vi "Big Variant Cluster.vi"(1 "Cluster":T1={"Variant"=variant(u32 0), "Variant 2"=variant(u32 0), "Variant 3"=variant(u32 0), "Variant 4"=variant(u32 0), "Variant 5"=variant(u32 0), "Variant 6"=variant(u32 0), "Variant 7"=variant(u32 0), "Variant 8"=variant(u32 0), "Variant 9"=variant(u32 0), "Variant 10"=variant(u32 0), "Variant 11"=variant(u32 0), "Variant 12"=variant(u32 0), "Variant 13"=variant(u32 0), "Variant 14"=variant(u32 0), "Variant 15"=variant(u32 0), "Variant 16"=variant(u32 0), "Variant 17"=variant(u32 0), "Variant 18"=variant(u32 0), "Variant 19"=variant(u32 0), "Variant 20"=variant(u32 0), "Variant 21"=variant(u32 0), "Variant 22"=variant(u32 0), "Variant 23"=variant(u32 0), "Variant 24"=variant(u32 0), "Variant 25"=variant(u32 0), "Variant 26"=variant(u32 0), "Variant 27"=variant(u32 0), "Variant 28"=variant(u32 0), "Variant 29"=variant(u32 0), "Variant 30"=variant(u32 0), "Variant 31"=variant(u32 0), "Variant 32"=variant(u32 0), "Variant 33"=variant(u32 0), "Variant 34"=variant(u32 0), "Variant 35"=variant(u32 0), "Variant 36"=variant(u32 0), "Variant 37"=variant(u32 0), "Variant 38"=variant(u32 0), "Variant 39"=variant(u32 0), "Variant 40"=variant(u32 0), "Variant 41"=variant(u32 0), "Variant 42"=variant(u32 0), "Variant 43"=variant(u32 0), "Variant 44"=variant(u32 0), "Variant 45"=variant(u32 0), "Variant 46"=variant(u32 0), "Variant 47"=variant(u32 0), "Variant 48"=variant(u32 0), "Variant 49"=variant(u32 0), "Variant 50"=variant(u32 0), "Variant 51"=variant(u32 0), "Variant 52"=variant(u32 0), "Variant 53"=variant(u32 0), "Variant 54"=variant(u32 0), "Variant 55"=variant(u32 0), "Variant 56"=variant(u32 0), "Variant 57"=variant(u32 0), "Variant 58"=variant(u32 0), "Variant 59"=variant(u32 0), "Variant 60"=variant(u32 0), "Variant 61"=variant(u32 0), "Variant 62"=variant(u32 0), "Variant 63"=variant(u32 0), "Variant 64"=variant(u32 0), "Variant 65"=variant(u32 0), "Variant 66"=variant(u32 0), "Variant 67"=variant(u32 0), "Variant 68"=variant(u32 0), "Variant 69"=variant(u32 0), "Variant 70"=variant(u32 0), "Variant 71"=variant(u32 0), "Variant 72"=variant(u32 0), "Variant 73"=variant(u32 0), "Variant 74"=variant(u32 0), "Variant 75"=variant(u32 0), "Variant 76"=variant(u32 0), "Variant 77"=variant(u32 0), "Variant 78"=variant(u32 0), "Variant 79"=variant(u32 0), "Variant 80"=variant(u32 0), "Variant 81"=variant(u32 0), "Variant 82"=variant(u32 0), "Variant 83"=variant(u32 0), "Variant 84"=variant(u32 0), "Variant 85"=variant(u32 0), "Variant 86"=variant(u32 0), "Variant 87"=variant(u32 0), "Variant 88"=variant(u32 0), "Variant 89"=variant(u32 0), "Variant 90"=variant(u32 0), "Variant 91"=variant(u32 0), "Variant 92"=variant(u32 0), "Variant 93"=variant(u32 0), "Variant 94"=variant(u32 0), "Variant 95"=variant(u32 0), "Variant 96"=variant(u32 0), "Variant 97"=variant(u32 0), "Variant 98"=variant(u32 0), "Variant 99"=variant(u32 0), "Variant 100"=variant(u32 0), "Variant 101"=variant(u32 0), "Variant 102"=variant(u32 0), "Variant 103"=variant(u32 0), "Variant 104"=variant(u32 0), "Variant 105"=variant(u32 0), "Variant 106"=variant(u32 0), "Variant 107"=variant(u32 0), "Variant 108"=variant(u32 0), "Variant 109"=variant(u32 0), "Variant 110"=variant(u32 0), "Variant 111"=variant(u32 0), "Variant 112"=variant(u32 0), "Variant 113"=variant(u32 0), "Variant 114"=variant(u32 0), "Variant 115"=variant(u32 0), "Variant 116"=variant(u32 0), "Variant 117"=variant(u32 0), "Variant 118"=variant(u32 0), "Variant 119"=variant(u32 0), "Variant 120"=variant(u32 0), "Variant 121"=variant(u32 0), "Variant 122"=variant(u32 0), "Variant 123"=variant(u32 0), "Variant 124"=variant(u32 0), "Variant 125"=variant(u32 0), "Variant 126"=variant(u32 0), "Variant 127"=variant(u32 0), "Variant 128"=variant(u32 0), "Variant 129"=variant(u32 0), "Variant 130"=variant(u32 0), "Variant 131"=variant(u32 0), "Variant 132"=variant(u32 0), "Variant 133"=variant(u32 0), "Variant 134"=variant(u32 0), "Variant 135"=variant(u32 0), "Variant 136"=variant(u32 0), "Variant 137"=variant(u32 0), "Variant 138"=variant(u32 0), "Variant 139"=variant(u32 0), "Variant 140"=variant(u32 0), "Variant 141"=variant(u32 0), "Variant 142"=variant(u32 0), "Variant 143"=variant(u32 0), "Variant 144"=variant(u32 0), "Variant 145"=variant(u32 0), "Variant 146"=variant(u32 0), "Variant 147"=variant(u32 0), "Variant 148"=variant(u32 0), "Variant 149"=variant(u32 0), "Variant 150"=variant(u32 0), "Variant 151"=variant(u32 0), "Variant 152"=variant(u32 0), "Variant 153"=variant(u32 0), "Variant 154"=variant(u32 0), "Variant 155"=variant(u32 0), "Variant 156"=variant(u32 0), "Variant 157"=variant(u32 0), "Variant 158"=variant(u32 0), "Variant 159"=variant(u32 0), "Variant 160"=variant(u32 0), "Variant 161"=variant(u32 0), "Variant 162"=variant(u32 0), "Variant 163"=variant(u32 0), "Variant 164"=variant(u32 0), "Variant 165"=variant(u32 0), "Variant 166"=variant(u32 0), "Variant 167"=variant(u32 0), "Variant 168"=variant(u32 0), "Variant 169"=variant(u32 0), "Variant 170"=variant(u32 0), "Variant 171"=variant(u32 0), "Variant 172"=variant(u32 0), "Variant 173"=variant(u32 0), "Variant 174"=variant(u32 0), "Variant 175"=variant(u32 0), "Variant 176"=variant(u32 0), "Variant 177"=variant(u32 0), "Variant 178"=variant(u32 0), "Variant 179"=variant(u32 0), "Variant 180"=variant(u32 0), "Variant 181"=variant(u32 0), "Variant 182"=variant(u32 0), "Variant 183"=variant(u32 0), "Variant 184"=variant(u32 0), "Variant 185"=variant(u32 0), "Variant 186"=variant(u32 0), "Variant 187"=variant(u32 0), "Variant 188"=variant(u32 0), "Variant 189"=variant(u32 0), "Variant 190"=variant(u32 0), "Variant 191"=variant(u32 0), "Variant 192"=variant(u32 0), "Variant 193"=variant(u32 0), "Variant 194"=variant(u32 0), "Variant 195"=variant(u32 0), "Variant 196"=variant(u32 0), "Variant 197"=variant(u32 0), "Variant 198"=variant(u32 0), "Variant 199"=variant(u32 0), "Variant 200"=variant(u32 0), "Variant 201"=variant(u32 0), "Variant 202"=variant(u32 0), "Variant 203"=variant(u32 0), "Variant 204"=variant(u32 0), "Variant 205"=variant(u32 0), "Variant 206"=variant(u32 0), "Variant 207"=variant(u32 0), "Variant 208"=variant(u32 0), "Variant 209"=variant(u32 0), "Variant 210"=variant(u32 0), "Variant 211"=variant(u32 0), "Variant 212"=variant(u32 0), "Variant 213"=variant(u32 0), "Variant 214"=variant(u32 0), "Variant 215"=variant(u32 0), "Variant 216"=variant(u32 0), "Variant 217"=variant(u32 0), "Variant 218"=variant(u32 0), "Variant 219"=variant(u32 0), "Variant 220"=variant(u32 0), "Variant 221"=variant(u32 0), "Variant 222"=variant(u32 0), "Variant 223"=variant(u32 0), "Variant 224"=variant(u32 0), "Variant 225"=variant(u32 0), "Variant 226"=variant(u32 0), "Variant 227"=variant(u32 0), "Variant 228"=variant(u32 0), "Variant 229"=variant(u32 0), "Variant 230"=variant(u32 0), "Variant 231"=variant(u32 0), "Variant 232"=variant(u32 0), "Variant 233"=variant(u32 0), "Variant 234"=variant(u32 0), "Variant 235"=variant(u32 0), "Variant 236"=variant(u32 0), "Variant 237"=variant(u32 0), "Variant 238"=variant(u32 0), "Variant 239"=variant(u32 0), "Variant 240"=variant(u32 0), "Variant 241"=variant(u32 0), "Variant 242"=variant(u32 0), "Variant 243"=variant(u32 0), "Variant 244"=variant(u32 0), "Variant 245"=variant(u32 0), "Variant 246"=variant(u32 0), "Variant 247"=variant(u32 0), "Variant 248"=variant(u32 0), "Variant 249"=variant(u32 0), "Variant 250"=variant(u32 0), "Variant 251"=variant(u32 0), "Variant 252"=variant(u32 0), "Variant 253"=variant(u32 0), "Variant 254"=variant(u32 0), "Variant 255"=variant(u32 0), "Variant 256"=variant(u32 0), "Variant 257"=variant(u32 0), "Variant 258"=variant(u32 0), "Variant 259"=variant(u32 0), "Variant 260"=variant(u32 0), "Variant 261"=variant(u32 0), "Variant 262"=variant(u32 0), "Variant 263"=variant(u32 0), "Variant 264"=variant(u32 0), "Variant 265"=variant(u32 0), "Variant 266"=variant(u32 0), "Variant 267"=variant(u32 0), "Variant 268"=variant(u32 0), "Variant 269"=variant(u32 0), "Variant 270"=variant(u32 0), "Variant 271"=variant(u32 0), "Variant 272"=variant(u32 0), "Variant 273"=variant(u32 0), "Variant 274"=variant(u32 0), "Variant 275"=variant(u32 0), "Variant 276"=variant(u32 0), "Variant 277"=variant(u32 0), "Variant 278"=variant(u32 0), "Variant 279"=variant(u32 0), "Variant 280"=variant(u32 0), "Variant 281"=variant(u32 0), "Variant 282"=variant(u32 0), "Variant 283"=variant(u32 0), "Variant 284"=variant(u32 0), "Variant 285"=variant(u32 0), "Variant 286"=variant(u32 0), "Variant 287"=variant(u32 0), "Variant 288"=variant(u32 0), "Variant 289"=variant(u32 0), "Variant 290"=variant(u32 0), "Variant 291"=variant(u32 0), "Variant 292"=variant(u32 0), "Variant 293"=variant(u32 0), "Variant 294"=variant(u32 0), "Variant 295"=variant(u32 0), "Variant 296"=variant(u32 0), "Variant 297"=variant(u32 0), "Variant 298"=variant(u32 0), "Variant 299"=variant(u32 0), "Variant 300"=variant(u32 0), "Variant 301"=variant(u32 0), "Variant 302"=variant(u32 0), "Variant 303"=variant(u32 0), "Variant 304"=variant(u32 0), "Variant 305"=variant(u32 0), "Variant 306"=variant(u32 0), "Variant 307"=variant(u32 0), "Variant 308"=variant(u32 0), "Variant 309"=variant(u32 0), "Variant 310"=variant(u32 0), "Variant 311"=variant(u32 0), "Variant 312"=variant(u32 0), "Variant 313"=variant(u32 0), "Variant 314"=variant(u32 0), "Variant 315"=variant(u32 0), "Variant 316"=variant(u32 0), "Variant 317"=variant(u32 0), "Variant 318"=variant(u32 0), "Variant 319"=variant(u32 0), "Variant 320"=variant(u32 0), "Variant 321"=variant(u32 0), "Variant 322"=variant(u32 0), "Variant 323"=variant(u32 0), "Variant 324"=variant(u32 0), "Variant 325"=variant(u32 0), "Variant 326"=variant(u32 0), "Variant 327"=variant(u32 0), "Variant 328"=variant(u32 0), "Variant 329"=variant(u32 0), "Variant 330"=variant(u32 0), "Variant 331"=variant(u32 0), "Variant 332"=variant(u32 0), "Variant 333"=variant(u32 0), "Variant 334"=variant(u32 0), "Variant 335"=variant(u32 0), "Variant 336"=variant(u32 0), "Variant 337"=variant(u32 0), "Variant 338"=variant(u32 0), "Variant 339"=variant(u32 0), "Variant 340"=variant(u32 0), "Variant 341"=variant(u32 0), "Variant 342"=variant(u32 0), "Variant 343"=variant(u32 0), "Variant 344"=variant(u32 0), "Variant 345"=variant(u32 0), "Variant 346"=variant(u32 0), "Variant 347"=variant(u32 0), "Variant 348"=variant(u32 0), "Variant 349"=variant(u32 0), "Variant 350"=variant(u32 0), "Variant 351"=variant(u32 0), "Variant 352"=variant(u32 0), "Variant 353"=variant(u32 0), "Variant 354"=variant(u32 0), "Variant 355"=variant(u32 0), "Variant 356"=variant(u32 0), "Variant 357"=variant(u32 0), "Variant 358"=variant(u32 0), "Variant 359"=variant(u32 0), "Variant 360"=variant(u32 0), "Variant 361"=variant(u32 0), "Variant 362"=variant(u32 0), "Variant 363"=variant(u32 0), "Variant 364"=variant(u32 0), "Variant 365"=variant(u32 0), "Variant 366"=variant(u32 0), "Variant 367"=variant(u32 0), "Variant 368"=variant(u32 0), "Variant 369"=variant(u32 0), "Variant 370"=variant(u32 0), "Variant 371"=variant(u32 0), "Variant 372"=variant(u32 0), "Variant 373"=variant(u32 0), "Variant 374"=variant(u32 0), "Variant 375"=variant(u32 0), "Variant 376"=variant(u32 0), "Variant 377"=variant(u32 0), "Variant 378"=variant(u32 0), "Variant 379"=variant(u32 0), "Variant 380"=variant(u32 0), "Variant 381"=variant(u32 0), "Variant 382"=variant(u32 0), "Variant 383"=variant(u32 0), "Variant 384"=variant(u32 0), "Variant 385"=variant(u32 0), "Variant 386"=variant(u32 0), "Variant 387"=variant(u32 0), "Variant 388"=variant(u32 0), "Variant 389"=variant(u32 0), "Variant 390"=variant(u32 0), "Variant 391"=variant(u32 0), "Variant 392"=variant(u32 0), "Variant 393"=variant(u32 0), "Variant 394"=variant(u32 0), "Variant 395"=variant(u32 0), "Variant 396"=variant(u32 0), "Variant 397"=variant(u32 0), "Variant 398"=variant(u32 0), "Variant 399"=variant(u32 0), "Variant 400"=variant(u32 0), "Variant 401"=variant(u32 0), "Variant 402"=variant(u32 0), "Variant 403"=variant(u32 0), "Variant 404"=variant(u32 0), "Variant 405"=variant(u32 0), "Variant 406"=variant(u32 0), "Variant 407"=variant(u32 0), "Variant 408"=variant(u32 0), "Variant 409"=variant(u32 0), "Variant 410"=variant(u32 0), "Variant 411"=variant(u32 0), "Variant 412"=variant(u32 0), "Variant 413"=variant(u32 0), "Variant 414"=variant(u32 0), "Variant 415"=variant(u32 0), "Variant 416"=variant(u32 0), "Variant 417"=variant(u32 0), "Variant 418"=variant(u32 0), "Variant 419"=variant(u32 0), "Variant 420"=variant(u32 0), "Variant 421"=variant(u32 0), "Variant 422"=variant(u32 0), "Variant 423"=variant(u32 0), "Variant 424"=variant(u32 0), "Variant 425"=variant(u32 0), "Variant 426"=variant(u32 0), "Variant 427"=variant(u32 0), "Variant 428"=variant(u32 0), "Variant 429"=variant(u32 0), "Variant 430"=variant(u32 0), "Variant 431"=variant(u32 0), "Variant 432"=variant(u32 0), "Variant 433"=variant(u32 0), "Variant 434"=variant(u32 0), "Variant 435"=variant(u32 0), "Variant 436"=variant(u32 0), "Variant 437"=variant(u32 0), "Variant 438"=variant(u32 0), "Variant 439"=variant(u32 0), "Variant 440"=variant(u32 0), "Variant 441"=variant(u32 0), "Variant 442"=variant(u32 0), "Variant 443"=variant(u32 0), "Variant 444"=variant(u32 0), "Variant 445"=variant(u32 0), "Variant 446"=variant(u32 0), "Variant 447"=variant(u32 0), "Variant 448"=variant(u32 0), "Variant 449"=variant(u32 0), "Variant 450"=variant(u32 0), "Variant 451"=variant(u32 0), "Variant 452"=variant(u32 0), "Variant 453"=variant(u32 0), "Variant 454"=variant(u32 0), "Variant 455"=variant(u32 0), "Variant 456"=variant(u32 0), "Variant 457"=variant(u32 0), "Variant 458"=variant(u32 0), "Variant 459"=variant(u32 0), "Variant 460"=variant(u32 0), "Variant 461"=variant(u32 0), "Variant 462"=variant(u32 0), "Variant 463"=variant(u32 0), "Variant 464"=variant(u32 0), "Variant 465"=variant(u32 0), "Variant 466"=variant(u32 0), "Variant 467"=variant(u32 0), "Variant 468"=variant(u32 0), "Variant 469"=variant(u32 0), "Variant 470"=variant(u32 0), "Variant 471"=variant(u32 0), "Variant 472"=variant(u32 0), "Variant 473"=variant(u32 0), "Variant 474"=variant(u32 0), "Variant 475"=variant(u32 0), "Variant 476"=variant(u32 0), "Variant 477"=variant(u32 0), "Variant 478"=variant(u32 0), "Variant 479"=variant(u32 0), "Variant 480"=variant(u32 0), "Variant 481"=variant(u32 0), "Variant 482"=variant(u32 0), "Variant 483"=variant(u32 0), "Variant 484"=variant(u32 0), "Variant 485"=variant(u32 0), "Variant 486"=variant(u32 0), "Variant 487"=variant(u32 0), "Variant 488"=variant(u32 0), "Variant 489"=variant(u32 0), "Variant 490"=variant(u32 0), "Variant 491"=variant(u32 0), "Variant 492"=variant(u32 0), "Variant 493"=variant(u32 0), "Variant 494"=variant(u32 0), "Variant 495"=variant(u32 0), "Variant 496"=variant(u32 0), "Variant 497"=variant(u32 0), "Variant 498"=variant(u32 0), "Variant 499"=variant(u32 0), "Variant 500"=variant(u32 0), "Variant 501"=variant(u32 0), "Variant 502"=variant(u32 0), "Variant 503"=variant(u32 0), "Variant 504"=variant(u32 0), "Variant 505"=variant(u32 0), "Variant 506"=variant(u32 0), "Variant 507"=variant(u32 0), "Variant 508"=variant(u32 0), "Variant 509"=variant(u32 0), "Variant 510"=variant(u32 0), "Variant 511"=variant(u32 0), "Variant 512"=variant(u32 0), "Variant 513"=variant(u32 0), "Variant 514"=variant(u32 0), "Variant 515"=variant(u32 0), "Variant 516"=variant(u32 0), "Variant 517"=variant(u32 0), "Variant 518"=variant(u32 0), "Variant 519"=variant(u32 0), "Variant 520"=variant(u32 0), "Variant 521"=variant(u32 0), "Variant 522"=variant(u32 0), "Variant 523"=variant(u32 0), "Variant 524"=variant(u32 0), "Variant 525"=variant(u32 0), "Variant 526"=variant(u32 0), "Variant 527"=variant(u32 0), "Variant 528"=variant(u32 0), "Variant 529"=variant(u32 0), "Variant 530"=variant(u32 0), "Variant 531"=variant(u32 0), "Variant 532"=variant(u32 0), "Variant 533"=variant(u32 0), "Variant 534"=variant(u32 0), "Variant 535"=variant(u32 0), "Variant 536"=variant(u32 0), "Variant 537"=variant(u32 0), "Variant 538"=variant(u32 0), "Variant 539"=variant(u32 0), "Variant 540"=variant(u32 0), "Variant 541"=variant(u32 0), "Variant 542"=variant(u32 0), "Variant 543"=variant(u32 0), "Variant 544"=variant(u32 0), "Variant 545"=variant(u32 0), "Variant 546"=variant(u32 0), "Variant 547"=variant(u32 0), "Variant 548"=variant(u32 0), "Variant 549"=variant(u32 0), "Variant 550"=variant(u32 0), "Variant 551"=variant(u32 0), "Variant 552"=variant(u32 0), "Variant 553"=variant(u32 0), "Variant 554"=variant(u32 0), "Variant 555"=variant(u32 0), "Variant 556"=variant(u32 0), "Variant 557"=variant(u32 0), "Variant 558"=variant(u32 0), "Variant 559"=variant(u32 0), "Variant 560"=variant(u32 0), "Variant 561"=variant(u32 0), "Variant 562"=variant(u32 0), "Variant 563"=variant(u32 0), "Variant 564"=variant(u32 0), "Variant 565"=variant(u32 0), "Variant 566"=variant(u32 0), "Variant 567"=variant(u32 0), "Variant 568"=variant(u32 0), "Variant 569"=variant(u32 0), "Variant 570"=variant(u32 0), "Variant 571"=variant(u32 0), "Variant 572"=variant(u32 0), "Variant 573"=variant(u32 0), "Variant 574"=variant(u32 0), "Variant 575"=variant(u32 0), "Variant 576"=variant(u32 0), "Variant 577"=variant(u32 0), "Variant 578"=variant(u32 0), "Variant 579"=variant(u32 0), "Variant 580"=variant(u32 0), "Variant 581"=variant(u32 0), "Variant 582"=variant(u32 0), "Variant 583"=variant(u32 0), "Variant 584"=variant(u32 0), "Variant 585"=variant(u32 0), "Variant 586"=variant(u32 0), "Variant 587"=variant(u32 0), "Variant 588"=variant(u32 0), "Variant 589"=variant(u32 0), "Variant 590"=variant(u32 0), "Variant 591"=variant(u32 0), "Variant 592"=variant(u32 0), "Variant 593"=variant(u32 0), "Variant 594"=variant(u32 0), "Variant 595"=variant(u32 0), "Variant 596"=variant(u32 0), "Variant 597"=variant(u32 0), "Variant 598"=variant(u32 0), "Variant 599"=variant(u32 0), "Variant 600"=variant(u32 0), "Variant 601"=variant(u32 0), "Variant 602"=variant(u32 0), "Variant 603"=variant(u32 0), "Variant 604"=variant(u32 0), "Variant 605"=variant(u32 0), "Variant 606"=variant(u32 0), "Variant 607"=variant(u32 0), "Variant 608"=variant(u32 0), "Variant 609"=variant(u32 0), "Variant 610"=variant(u32 0), "Variant 611"=variant(u32 0), "Variant 612"=variant(u32 0), "Variant 613"=variant(u32 0), "Variant 614"=variant(u32 0), "Variant 615"=variant(u32 0), "Variant 616"=variant(u32 0), "Variant 617"=variant(u32 0), "Variant 618"=variant(u32 0), "Variant 619"=variant(u32 0), "Variant 620"=variant(u32 0), "Variant 621"=variant(u32 0), "Variant 622"=variant(u32 0), "Variant 623"=variant(u32 0), "Variant 624"=variant(u32 0), "Variant 625"=variant(u32 0), "Variant 626"=variant(u32 0), "Variant 627"=variant(u32 0), "Variant 628"=variant(u32 0), "Variant 629"=variant(u32 0), "Variant 630"=variant(u32 0), "Variant 631"=variant(u32 0), "Variant 632"=variant(u32 0), "Variant 633"=variant(u32 0), "Variant 634"=variant(u32 0), "Variant 635"=variant(u32 0), "Variant 636"=variant(u32 0), "Variant 637"=variant(u32 0), "Variant 638"=variant(u32 0), "Variant 639"=variant(u32 0), "Variant 640"=variant(u32 0), "Variant 641"=variant(u32 0), "Variant 642"=variant(u32 0), "Variant 643"=variant(u32 0), "Variant 644"=variant(u32 0), "Variant 645"=variant(u32 0), "Variant 646"=variant(u32 0), "Variant 647"=variant(u32 0), "Variant 648"=variant(u32 0), "Variant 649"=variant(u32 0), "Variant 650"=variant(u32 0), "Variant 651"=variant(u32 0), "Variant 652"=variant(u32 0), "Variant 653"=variant(u32 0), "Variant 654"=variant(u32 0), "Variant 655"=variant(u32 0), "Variant 656"=variant(u32 0), "Variant 657"=variant(u32 0), "Variant 658"=variant(u32 0), "Variant 659"=variant(u32 0), "Variant 660"=variant(u32 0), "Variant 661"=variant(u32 0), "Variant 662"=variant(u32 0), "Variant 663"=variant(u32 0), "Variant 664"=variant(u32 0), "Variant 665"=variant(u32 0), "Variant 666"=variant(u32 0), "Variant 667"=variant(u32 0), "Variant 668"=variant(u32 0), "Variant 669"=variant(u32 0), "Variant 670"=variant(u32 0), "Variant 671"=variant(u32 0), "Variant 672"=variant(u32 0), "Variant 673"=variant(u32 0), "Variant 674"=variant(u32 0), "Variant 675"=variant(u32 0), "Variant 676"=variant(u32 0), "Variant 677"=variant(u32 0), "Variant 678"=variant(u32 0), "Variant 679"=variant(u32 0), "Variant 680"=variant(u32 0), "Variant 681"=variant(u32 0), "Variant 682"=variant(u32 0), "Variant 683"=variant(u32 0), "Variant 684"=variant(u32 0), "Variant 685"=variant(u32 0), "Variant 686"=variant(u32 0), "Variant 687"=variant(u32 0), "Variant 688"=variant(u32 0), "Variant 689"=variant(u32 0), "Variant 690"=variant(u32 0), "Variant 691"=variant(u32 0), "Variant 692"=variant(u32 0), "Variant 693"=variant(u32 0), "Variant 694"=variant(u32 0), "Variant 695"=variant(u32 0), "Variant 696"=variant(u32 0), "Variant 697"=variant(u32 0), "Variant 698"=variant(u32 0), "Variant 699"=variant(u32 0), "Variant 700"=variant(u32 0), "Variant 701"=variant(u32 0), "Variant 702"=variant(u32 0), "Variant 703"=variant(u32 0), "Variant 704"=variant(u32 0), "Variant 705"=variant(u32 0), "Variant 706"=variant(u32 0), "Variant 707"=variant(u32 0), "Variant 708"=variant(u32 0), "Variant 709"=variant(u32 0), "Variant 710"=variant(u32 0), "Variant 711"=variant(u32 0), "Variant 712"=variant(u32 0), "Variant 713"=variant(u32 0), "Variant 714"=variant(u32 0), "Variant 715"=variant(u32 0), "Variant 716"=variant(u32 0), "Variant 717"=variant(u32 0), "Variant 718"=variant(u32 0), "Variant 719"=variant(u32 0), "Variant 720"=variant(u32 0), "Variant 721"=variant(u32 0), "Variant 722"=variant(u32 0), "Variant 723"=variant(u32 0), "Variant 724"=variant(u32 0), "Variant 725"=variant(u32 0), "Variant 726"=variant(u32 0), "Variant 727"=variant(u32 0), "Variant 728"=variant(u32 0), "Variant 729"=variant(u32 0), "Variant 730"=variant(u32 0), "Variant 731"=variant(u32 0), "Variant 732"=variant(u32 0), "Variant 733"=variant(u32 0), "Variant 734"=variant(u32 0), "Variant 735"=variant(u32 0), "Variant 736"=variant(u32 0), "Variant 737"=variant(u32 0), "Variant 738"=variant(u32 0), "Variant 739"=variant(u32 0), "Variant 740"=variant(u32 0), "Variant 741"=variant(u32 0), "Variant 742"=variant(u32 0), "Variant 743"=variant(u32 0), "Variant 744"=variant(u32 0), "Variant 745"=variant(u32 0), "Variant 746"=variant(u32 0), "Variant 747"=variant(u32 0), "Variant 748"=variant(u32 0), "Variant 749"=variant(u32 0), "Variant 750"=variant(u32 0), "Variant 751"=variant(u32 0), "Variant 752"=variant(u32 0), "Variant 753"=variant(u32 0), "Variant 754"=variant(u32 0), "Variant 755"=variant(u32 0), "Variant 756"=variant(u32 0), "Variant 757"=variant(u32 0), "Variant 758"=variant(u32 0), "Variant 759"=variant(u32 0), "Variant 760"=variant(u32 0), "Variant 761"=variant(u32 0), "Variant 762"=variant(u32 0), "Variant 763"=variant(u32 0), "Variant 764"=variant(u32 0), "Variant 765"=variant(u32 0), "Variant 766"=variant(u32 0), "Variant 767"=variant(u32 0), "Variant 768"=variant(u32 0), "Variant 769"=variant(u32 0), "Variant 770"=variant(u32 0), "Variant 771"=variant(u32 0), "Variant 772"=variant(u32 0), "Variant 773"=variant(u32 0), "Variant 774"=variant(u32 0), "Variant 775"=variant(u32 0), "Variant 776"=variant(u32 0), "Variant 777"=variant(u32 0), "Variant 778"=variant(u32 0), "Variant 779"=variant(u32 0), "Variant 780"=variant(u32 0), "Variant 781"=variant(u32 0), "Variant 782"=variant(u32 0), "Variant 783"=variant(u32 0), "Variant 784"=variant(u32 0), "Variant 785"=variant(u32 0), "Variant 786"=variant(u32 0), "Variant 787"=variant(u32 0), "Variant 788"=variant(u32 0), "Variant 789"=variant(u32 0), "Variant 790"=variant(u32 0), "Variant 791"=variant(u32 0), "Variant 792"=variant(u32 0), "Variant 793"=variant(u32 0), "Variant 794"=variant(u32 0), "Variant 795"=variant(u32 0), "Variant 796"=variant(u32 0), "Variant 797"=variant(u32 0), "Variant 798"=variant(u32 0), "Variant 799"=variant(u32 0), "Variant 800"=variant(u32 0), "Variant 801"=variant(u32 0), "Variant 802"=variant(u32 0), "Variant 803"=variant(u32 0), "Variant 804"=variant(u32 0), "Variant 805"=variant(u32 0), "Variant 806"=variant(u32 0), "Variant 807"=variant(u32 0), "Variant 808"=variant(u32 0), "Variant 809"=variant(u32 0), "Variant 810"=variant(u32 0), "Variant 811"=variant(u32 0), "Variant 812"=variant(u32 0), "Variant 813"=variant(u32 0), "Variant 814"=variant(u32 0), "Variant 815"=variant(u32 0), "Variant 816"=variant(u32 0), "Variant 817"=variant(u32 0), "Variant 818"=variant(u32 0), "Variant 819"=variant(u32 0), "Variant 820"=variant(u32 0), "Variant 821"=variant(u32 0), "Variant 822"=variant(u32 0), "Variant 823"=variant(u32 0), "Variant 824"=variant(u32 0), "Variant 825"=variant(u32 0), "Variant 826"=variant(u32 0), "Variant 827"=variant(u32 0), "Variant 828"=variant(u32 0), "Variant 829"=variant(u32 0), "Variant 830"=variant(u32 0), "Variant 831"=variant(u32 0), "Variant 832"=variant(u32 0), "Variant 833"=variant(u32 0), "Variant 834"=variant(u32 0), "Variant 835"=variant(u32 0), "Variant 836"=variant(u32 0), "Variant 837"=variant(u32 0), "Variant 838"=variant(u32 0), "Variant 839"=variant(u32 0), "Variant 840"=variant(u32 0), "Variant 841"=variant(u32 0), "Variant 842"=variant(u32 0), "Variant 843"=variant(u32 0), "Variant 844"=variant(u32 0), "Variant 845"=variant(u32 0), "Variant 846"=variant(u32 0), "Variant 847"=variant(u32 0), "Variant 848"=variant(u32 0), "Variant 849"=variant(u32 0), "Variant 850"=variant(u32 0), "Variant 851"=variant(u32 0), "Variant 852"=variant(u32 0), "Variant 853"=variant(u32 0), "Variant 854"=variant(u32 0), "Variant 855"=variant(u32 0), "Variant 856"=variant(u32 0), "Variant 857"=variant(u32 0), "Variant 858"=variant(u32 0), "Variant 859"=variant(u32 0), "Variant 860"=variant(u32 0), "Variant 861"=variant(u32 0), "Variant 862"=variant(u32 0), "Variant 863"=variant(u32 0), "Variant 864"=variant(u32 0), "Variant 865"=variant(u32 0), "Variant 866"=variant(u32 0), "Variant 867"=variant(u32 0), "Variant 868"=variant(u32 0), "Variant 869"=variant(u32 0), "Variant 870"=variant(u32 0), "Variant 871"=variant(u32 0), "Variant 872"=variant(u32 0), "Variant 873"=variant(u32 0), "Variant 874"=variant(u32 0), "Variant 875"=variant(u32 0), "Variant 876"=variant(u32 0), "Variant 877"=variant(u32 0), "Variant 878"=variant(u32 0), "Variant 879"=variant(u32 0), "Variant 880"=variant(u32 0), "Variant 881"=variant(u32 0), "Variant 882"=variant(u32 0), "Variant 883"=variant(u32 0), "Variant 884"=variant(u32 0), "Variant 885"=variant(u32 0), "Variant 886"=variant(u32 0), "Variant 887"=variant(u32 0), "Variant 888"=variant(u32 0), "Variant 889"=variant(u32 0), "Variant 890"=variant(u32 0), "Variant 891"=variant(u32 0), "Variant 892"=variant(u32 0), "Variant 893"=variant(u32 0), "Variant 894"=variant(u32 0), "Variant 895"=variant(u32 0), "Variant 896"=variant(u32 0), "Variant 897"=variant(u32 0), "Variant 898"=variant(u32 0), "Variant 899"=variant(u32 0), "Variant 900"=variant(u32 0), "Variant 901"=variant(u32 0), "Variant 902"=variant(u32 0), "Variant 903"=variant(u32 0), "Variant 904"=variant(u32 0), "Variant 905"=variant(u32 0), "Variant 906"=variant(u32 0), "Variant 907"=variant(u32 0), "Variant 908"=variant(u32 0), "Variant 909"=variant(u32 0), "Variant 910"=variant(u32 0), "Variant 911"=variant(u32 0), "Variant 912"=variant(u32 0), "Variant 913"=variant(u32 0), "Variant 914"=variant(u32 0), "Variant 915"=variant(u32 0), "Variant 916"=variant(u32 0), "Variant 917"=variant(u32 0), "Variant 918"=variant(u32 0), "Variant 919"=variant(u32 0), "Variant 920"=variant(u32 0), "Variant 921"=variant(u32 0), "Variant 922"=variant(u32 0), "Variant 923"=variant(u32 0), "Variant 924"=variant(u32 0), "Variant 925"=variant(u32 0), "Variant 926"=variant(u32 0), "Variant 927"=variant(u32 0), "Variant 928"=variant(u32 0), "Variant 929"=variant(u32 0), "Variant 930"=variant(u32 0), "Variant 931"=variant(u32 0), "Variant 932"=variant(u32 0), "Variant 933"=variant(u32 0), "Variant 934"=variant(u32 0), "Variant 935"=variant(u32 0), "Variant 936"=variant(u32 0), "Variant 937"=variant(u32 0), "Variant 938"=variant(u32 0), "Variant 939"=variant(u32 0), "Variant 940"=variant(u32 0), "Variant 941"=variant(u32 0), "Variant 942"=variant(u32 0), "Variant 943"=variant(u32 0), "Variant 944"=variant(u32 0), "Variant 945"=variant(u32 0), "Variant 946"=variant(u32 0), "Variant 947"=variant(u32 0), "Variant 948"=variant(u32 0), "Variant 949"=variant(u32 0), "Variant 950"=variant(u32 0), "Variant 951"=variant(u32 0), "Variant 952"=variant(u32 0), "Variant 953"=variant(u32 0), "Variant 954"=variant(u32 0), "Variant 955"=variant(u32 0), "Variant 956"=variant(u32 0), "Variant 957"=variant(u32 0), "Variant 958"=variant(u32 0), "Variant 959"=variant(u32 0), "Variant 960"=variant(u32 0), "Variant 961"=variant(u32 0), "Variant 962"=variant(u32 0), "Variant 963"=variant(u32 0), "Variant 964"=variant(u32 0), "Variant 965"=variant(u32 0), "Variant 966"=variant(u32 0), "Variant 967"=variant(u32 0), "Variant 968"=variant(u32 0), "Variant 969"=variant(u32 0), "Variant 970"=variant(u32 0), "Variant 971"=variant(u32 0), "Variant 972"=variant(u32 0), "Variant 973"=variant(u32 0), "Variant 974"=variant(u32 0), "Variant 975"=variant(u32 0), "Variant 976"=variant(u32 0), "Variant 977"=variant(u32 0), "Variant 978"=variant(u32 0), "Variant 979"=variant(u32 0), "Variant 980"=variant(u32 0), "Variant 981"=variant(u32 0), "Variant 982"=variant(u32 0), "Variant 983"=variant(u32 0), "Variant 984"=variant(u32 0), "Variant 985"=variant(u32 0), "Variant 986"=variant(u32 0), "Variant 987"=variant(u32 0), "Variant 988"=variant(u32 0), "Variant 989"=variant(u32 0), "Variant 990"=variant(u32 0), "Variant 991"=variant(u32 0), "Variant 992"=variant(u32 0), "Variant 993"=variant(u32 0), "Variant 994"=variant(u32 0), "Variant 995"=variant(u32 0), "Variant 996"=variant(u32 0), "Variant 997"=variant(u32 0), "Variant 998"=variant(u32 0), "Variant 999"=variant(u32 0), "Variant 1000"=variant(u32 123)}) -> (0 "Cluster 2":T1)   [LabVIEW 2012]
types:
  T1 = cluster{"Variant":variant, "Variant 2":variant, "Variant 3":variant, "Variant 4":variant, "Variant 5":variant, "Variant 6":variant, "Variant 7":variant, "Variant 8":variant, "Variant 9":variant, "Variant 10":variant, "Variant 11":variant, "Variant 12":variant, "Variant 13":variant, "Variant 14":variant, "Variant 15":variant, "Variant 16":variant, "Variant 17":variant, "Variant 18":variant, "Variant 19":variant, "Variant 20":variant, "Variant 21":variant, "Variant 22":variant, "Variant 23":variant, "Variant 24":variant, "Variant 25":variant, "Variant 26":variant, "Variant 27":variant, "Variant 28":variant, "Variant 29":variant, "Variant 30":variant, "Variant 31":variant, "Variant 32":variant, "Variant 33":variant, "Variant 34":variant, "Variant 35":variant, "Variant 36":variant, "Variant 37":variant, "Variant 38":variant, "Variant 39":variant, "Variant 40":variant, "Variant 41":variant, "Variant 42":variant, "Variant 43":variant, "Variant 44":variant, "Variant 45":variant, "Variant 46":variant, "Variant 47":variant, "Variant 48":variant, "Variant 49":variant, "Variant 50":variant, "Variant 51":variant, "Variant 52":variant, "Variant 53":variant, "Variant 54":variant, "Variant 55":variant, "Variant 56":variant, "Variant 57":variant, "Variant 58":variant, "Variant 59":variant, "Variant 60":variant, "Variant 61":variant, "Variant 62":variant, "Variant 63":variant, "Variant 64":variant, "Variant 65":variant, "Variant 66":variant, "Variant 67":variant, "Variant 68":variant, "Variant 69":variant, "Variant 70":variant, "Variant 71":variant, "Variant 72":variant, "Variant 73":variant, "Variant 74":variant, "Variant 75":variant, "Variant 76":variant, "Variant 77":variant, "Variant 78":variant, "Variant 79":variant, "Variant 80":variant, "Variant 81":variant, "Variant 82":variant, "Variant 83":variant, "Variant 84":variant, "Variant 85":variant, "Variant 86":variant, "Variant 87":variant, "Variant 88":variant, "Variant 89":variant, "Variant 90":variant, "Variant 91":variant, "Variant 92":variant, "Variant 93":variant, "Variant 94":variant, "Variant 95":variant, "Variant 96":variant, "Variant 97":variant, "Variant 98":variant, "Variant 99":variant, "Variant 100":variant, "Variant 101":variant, "Variant 102":variant, "Variant 103":variant, "Variant 104":variant, "Variant 105":variant, "Variant 106":variant, "Variant 107":variant, "Variant 108":variant, "Variant 109":variant, "Variant 110":variant, "Variant 111":variant, "Variant 112":variant, "Variant 113":variant, "Variant 114":variant, "Variant 115":variant, "Variant 116":variant, "Variant 117":variant, "Variant 118":variant, "Variant 119":variant, "Variant 120":variant, "Variant 121":variant, "Variant 122":variant, "Variant 123":variant, "Variant 124":variant, "Variant 125":variant, "Variant 126":variant, "Variant 127":variant, "Variant 128":variant, "Variant 129":variant, "Variant 130":variant, "Variant 131":variant, "Variant 132":variant, "Variant 133":variant, "Variant 134":variant, "Variant 135":variant, "Variant 136":variant, "Variant 137":variant, "Variant 138":variant, "Variant 139":variant, "Variant 140":variant, "Variant 141":variant, "Variant 142":variant, "Variant 143":variant, "Variant 144":variant, "Variant 145":variant, "Variant 146":variant, "Variant 147":variant, "Variant 148":variant, "Variant 149":variant, "Variant 150":variant, "Variant 151":variant, "Variant 152":variant, "Variant 153":variant, "Variant 154":variant, "Variant 155":variant, "Variant 156":variant, "Variant 157":variant, "Variant 158":variant, "Variant 159":variant, "Variant 160":variant, "Variant 161":variant, "Variant 162":variant, "Variant 163":variant, "Variant 164":variant, "Variant 165":variant, "Variant 166":variant, "Variant 167":variant, "Variant 168":variant, "Variant 169":variant, "Variant 170":variant, "Variant 171":variant, "Variant 172":variant, "Variant 173":variant, "Variant 174":variant, "Variant 175":variant, "Variant 176":variant, "Variant 177":variant, "Variant 178":variant, "Variant 179":variant, "Variant 180":variant, "Variant 181":variant, "Variant 182":variant, "Variant 183":variant, "Variant 184":variant, "Variant 185":variant, "Variant 186":variant, "Variant 187":variant, "Variant 188":variant, "Variant 189":variant, "Variant 190":variant, "Variant 191":variant, "Variant 192":variant, "Variant 193":variant, "Variant 194":variant, "Variant 195":variant, "Variant 196":variant, "Variant 197":variant, "Variant 198":variant, "Variant 199":variant, "Variant 200":variant, "Variant 201":variant, "Variant 202":variant, "Variant 203":variant, "Variant 204":variant, "Variant 205":variant, "Variant 206":variant, "Variant 207":variant, "Variant 208":variant, "Variant 209":variant, "Variant 210":variant, "Variant 211":variant, "Variant 212":variant, "Variant 213":variant, "Variant 214":variant, "Variant 215":variant, "Variant 216":variant, "Variant 217":variant, "Variant 218":variant, "Variant 219":variant, "Variant 220":variant, "Variant 221":variant, "Variant 222":variant, "Variant 223":variant, "Variant 224":variant, "Variant 225":variant, "Variant 226":variant, "Variant 227":variant, "Variant 228":variant, "Variant 229":variant, "Variant 230":variant, "Variant 231":variant, "Variant 232":variant, "Variant 233":variant, "Variant 234":variant, "Variant 235":variant, "Variant 236":variant, "Variant 237":variant, "Variant 238":variant, "Variant 239":variant, "Variant 240":variant, "Variant 241":variant, "Variant 242":variant, "Variant 243":variant, "Variant 244":variant, "Variant 245":variant, "Variant 246":variant, "Variant 247":variant, "Variant 248":variant, "Variant 249":variant, "Variant 250":variant, "Variant 251":variant, "Variant 252":variant, "Variant 253":variant, "Variant 254":variant, "Variant 255":variant, "Variant 256":variant, "Variant 257":variant, "Variant 258":variant, "Variant 259":variant, "Variant 260":variant, "Variant 261":variant, "Variant 262":variant, "Variant 263":variant, "Variant 264":variant, "Variant 265":variant, "Variant 266":variant, "Variant 267":variant, "Variant 268":variant, "Variant 269":variant, "Variant 270":variant, "Variant 271":variant, "Variant 272":variant, "Variant 273":variant, "Variant 274":variant, "Variant 275":variant, "Variant 276":variant, "Variant 277":variant, "Variant 278":variant, "Variant 279":variant, "Variant 280":variant, "Variant 281":variant, "Variant 282":variant, "Variant 283":variant, "Variant 284":variant, "Variant 285":variant, "Variant 286":variant, "Variant 287":variant, "Variant 288":variant, "Variant 289":variant, "Variant 290":variant, "Variant 291":variant, "Variant 292":variant, "Variant 293":variant, "Variant 294":variant, "Variant 295":variant, "Variant 296":variant, "Variant 297":variant, "Variant 298":variant, "Variant 299":variant, "Variant 300":variant, "Variant 301":variant, "Variant 302":variant, "Variant 303":variant, "Variant 304":variant, "Variant 305":variant, "Variant 306":variant, "Variant 307":variant, "Variant 308":variant, "Variant 309":variant, "Variant 310":variant, "Variant 311":variant, "Variant 312":variant, "Variant 313":variant, "Variant 314":variant, "Variant 315":variant, "Variant 316":variant, "Variant 317":variant, "Variant 318":variant, "Variant 319":variant, "Variant 320":variant, "Variant 321":variant, "Variant 322":variant, "Variant 323":variant, "Variant 324":variant, "Variant 325":variant, "Variant 326":variant, "Variant 327":variant, "Variant 328":variant, "Variant 329":variant, "Variant 330":variant, "Variant 331":variant, "Variant 332":variant, "Variant 333":variant, "Variant 334":variant, "Variant 335":variant, "Variant 336":variant, "Variant 337":variant, "Variant 338":variant, "Variant 339":variant, "Variant 340":variant, "Variant 341":variant, "Variant 342":variant, "Variant 343":variant, "Variant 344":variant, "Variant 345":variant, "Variant 346":variant, "Variant 347":variant, "Variant 348":variant, "Variant 349":variant, "Variant 350":variant, "Variant 351":variant, "Variant 352":variant, "Variant 353":variant, "Variant 354":variant, "Variant 355":variant, "Variant 356":variant, "Variant 357":variant, "Variant 358":variant, "Variant 359":variant, "Variant 360":variant, "Variant 361":variant, "Variant 362":variant, "Variant 363":variant, "Variant 364":variant, "Variant 365":variant, "Variant 366":variant, "Variant 367":variant, "Variant 368":variant, "Variant 369":variant, "Variant 370":variant, "Variant 371":variant, "Variant 372":variant, "Variant 373":variant, "Variant 374":variant, "Variant 375":variant, "Variant 376":variant, "Variant 377":variant, "Variant 378":variant, "Variant 379":variant, "Variant 380":variant, "Variant 381":variant, "Variant 382":variant, "Variant 383":variant, "Variant 384":variant, "Variant 385":variant, "Variant 386":variant, "Variant 387":variant, "Variant 388":variant, "Variant 389":variant, "Variant 390":variant, "Variant 391":variant, "Variant 392":variant, "Variant 393":variant, "Variant 394":variant, "Variant 395":variant, "Variant 396":variant, "Variant 397":variant, "Variant 398":variant, "Variant 399":variant, "Variant 400":variant, "Variant 401":variant, "Variant 402":variant, "Variant 403":variant, "Variant 404":variant, "Variant 405":variant, "Variant 406":variant, "Variant 407":variant, "Variant 408":variant, "Variant 409":variant, "Variant 410":variant, "Variant 411":variant, "Variant 412":variant, "Variant 413":variant, "Variant 414":variant, "Variant 415":variant, "Variant 416":variant, "Variant 417":variant, "Variant 418":variant, "Variant 419":variant, "Variant 420":variant, "Variant 421":variant, "Variant 422":variant, "Variant 423":variant, "Variant 424":variant, "Variant 425":variant, "Variant 426":variant, "Variant 427":variant, "Variant 428":variant, "Variant 429":variant, "Variant 430":variant, "Variant 431":variant, "Variant 432":variant, "Variant 433":variant, "Variant 434":variant, "Variant 435":variant, "Variant 436":variant, "Variant 437":variant, "Variant 438":variant, "Variant 439":variant, "Variant 440":variant, "Variant 441":variant, "Variant 442":variant, "Variant 443":variant, "Variant 444":variant, "Variant 445":variant, "Variant 446":variant, "Variant 447":variant, "Variant 448":variant, "Variant 449":variant, "Variant 450":variant, "Variant 451":variant, "Variant 452":variant, "Variant 453":variant, "Variant 454":variant, "Variant 455":variant, "Variant 456":variant, "Variant 457":variant, "Variant 458":variant, "Variant 459":variant, "Variant 460":variant, "Variant 461":variant, "Variant 462":variant, "Variant 463":variant, "Variant 464":variant, "Variant 465":variant, "Variant 466":variant, "Variant 467":variant, "Variant 468":variant, "Variant 469":variant, "Variant 470":variant, "Variant 471":variant, "Variant 472":variant, "Variant 473":variant, "Variant 474":variant, "Variant 475":variant, "Variant 476":variant, "Variant 477":variant, "Variant 478":variant, "Variant 479":variant, "Variant 480":variant, "Variant 481":variant, "Variant 482":variant, "Variant 483":variant, "Variant 484":variant, "Variant 485":variant, "Variant 486":variant, "Variant 487":variant, "Variant 488":variant, "Variant 489":variant, "Variant 490":variant, "Variant 491":variant, "Variant 492":variant, "Variant 493":variant, "Variant 494":variant, "Variant 495":variant, "Variant 496":variant, "Variant 497":variant, "Variant 498":variant, "Variant 499":variant, "Variant 500":variant, "Variant 501":variant, "Variant 502":variant, "Variant 503":variant, "Variant 504":variant, "Variant 505":variant, "Variant 506":variant, "Variant 507":variant, "Variant 508":variant, "Variant 509":variant, "Variant 510":variant, "Variant 511":variant, "Variant 512":variant, "Variant 513":variant, "Variant 514":variant, "Variant 515":variant, "Variant 516":variant, "Variant 517":variant, "Variant 518":variant, "Variant 519":variant, "Variant 520":variant, "Variant 521":variant, "Variant 522":variant, "Variant 523":variant, "Variant 524":variant, "Variant 525":variant, "Variant 526":variant, "Variant 527":variant, "Variant 528":variant, "Variant 529":variant, "Variant 530":variant, "Variant 531":variant, "Variant 532":variant, "Variant 533":variant, "Variant 534":variant, "Variant 535":variant, "Variant 536":variant, "Variant 537":variant, "Variant 538":variant, "Variant 539":variant, "Variant 540":variant, "Variant 541":variant, "Variant 542":variant, "Variant 543":variant, "Variant 544":variant, "Variant 545":variant, "Variant 546":variant, "Variant 547":variant, "Variant 548":variant, "Variant 549":variant, "Variant 550":variant, "Variant 551":variant, "Variant 552":variant, "Variant 553":variant, "Variant 554":variant, "Variant 555":variant, "Variant 556":variant, "Variant 557":variant, "Variant 558":variant, "Variant 559":variant, "Variant 560":variant, "Variant 561":variant, "Variant 562":variant, "Variant 563":variant, "Variant 564":variant, "Variant 565":variant, "Variant 566":variant, "Variant 567":variant, "Variant 568":variant, "Variant 569":variant, "Variant 570":variant, "Variant 571":variant, "Variant 572":variant, "Variant 573":variant, "Variant 574":variant, "Variant 575":variant, "Variant 576":variant, "Variant 577":variant, "Variant 578":variant, "Variant 579":variant, "Variant 580":variant, "Variant 581":variant, "Variant 582":variant, "Variant 583":variant, "Variant 584":variant, "Variant 585":variant, "Variant 586":variant, "Variant 587":variant, "Variant 588":variant, "Variant 589":variant, "Variant 590":variant, "Variant 591":variant, "Variant 592":variant, "Variant 593":variant, "Variant 594":variant, "Variant 595":variant, "Variant 596":variant, "Variant 597":variant, "Variant 598":variant, "Variant 599":variant, "Variant 600":variant, "Variant 601":variant, "Variant 602":variant, "Variant 603":variant, "Variant 604":variant, "Variant 605":variant, "Variant 606":variant, "Variant 607":variant, "Variant 608":variant, "Variant 609":variant, "Variant 610":variant, "Variant 611":variant, "Variant 612":variant, "Variant 613":variant, "Variant 614":variant, "Variant 615":variant, "Variant 616":variant, "Variant 617":variant, "Variant 618":variant, "Variant 619":variant, "Variant 620":variant, "Variant 621":variant, "Variant 622":variant, "Variant 623":variant, "Variant 624":variant, "Variant 625":variant, "Variant 626":variant, "Variant 627":variant, "Variant 628":variant, "Variant 629":variant, "Variant 630":variant, "Variant 631":variant, "Variant 632":variant, "Variant 633":variant, "Variant 634":variant, "Variant 635":variant, "Variant 636":variant, "Variant 637":variant, "Variant 638":variant, "Variant 639":variant, "Variant 640":variant, "Variant 641":variant, "Variant 642":variant, "Variant 643":variant, "Variant 644":variant, "Variant 645":variant, "Variant 646":variant, "Variant 647":variant, "Variant 648":variant, "Variant 649":variant, "Variant 650":variant, "Variant 651":variant, "Variant 652":variant, "Variant 653":variant, "Variant 654":variant, "Variant 655":variant, "Variant 656":variant, "Variant 657":variant, "Variant 658":variant, "Variant 659":variant, "Variant 660":variant, "Variant 661":variant, "Variant 662":variant, "Variant 663":variant, "Variant 664":variant, "Variant 665":variant, "Variant 666":variant, "Variant 667":variant, "Variant 668":variant, "Variant 669":variant, "Variant 670":variant, "Variant 671":variant, "Variant 672":variant, "Variant 673":variant, "Variant 674":variant, "Variant 675":variant, "Variant 676":variant, "Variant 677":variant, "Variant 678":variant, "Variant 679":variant, "Variant 680":variant, "Variant 681":variant, "Variant 682":variant, "Variant 683":variant, "Variant 684":variant, "Variant 685":variant, "Variant 686":variant, "Variant 687":variant, "Variant 688":variant, "Variant 689":variant, "Variant 690":variant, "Variant 691":variant, "Variant 692":variant, "Variant 693":variant, "Variant 694":variant, "Variant 695":variant, "Variant 696":variant, "Variant 697":variant, "Variant 698":variant, "Variant 699":variant, "Variant 700":variant, "Variant 701":variant, "Variant 702":variant, "Variant 703":variant, "Variant 704":variant, "Variant 705":variant, "Variant 706":variant, "Variant 707":variant, "Variant 708":variant, "Variant 709":variant, "Variant 710":variant, "Variant 711":variant, "Variant 712":variant, "Variant 713":variant, "Variant 714":variant, "Variant 715":variant, "Variant 716":variant, "Variant 717":variant, "Variant 718":variant, "Variant 719":variant, "Variant 720":variant, "Variant 721":variant, "Variant 722":variant, "Variant 723":variant, "Variant 724":variant, "Variant 725":variant, "Variant 726":variant, "Variant 727":variant, "Variant 728":variant, "Variant 729":variant, "Variant 730":variant, "Variant 731":variant, "Variant 732":variant, "Variant 733":variant, "Variant 734":variant, "Variant 735":variant, "Variant 736":variant, "Variant 737":variant, "Variant 738":variant, "Variant 739":variant, "Variant 740":variant, "Variant 741":variant, "Variant 742":variant, "Variant 743":variant, "Variant 744":variant, "Variant 745":variant, "Variant 746":variant, "Variant 747":variant, "Variant 748":variant, "Variant 749":variant, "Variant 750":variant, "Variant 751":variant, "Variant 752":variant, "Variant 753":variant, "Variant 754":variant, "Variant 755":variant, "Variant 756":variant, "Variant 757":variant, "Variant 758":variant, "Variant 759":variant, "Variant 760":variant, "Variant 761":variant, "Variant 762":variant, "Variant 763":variant, "Variant 764":variant, "Variant 765":variant, "Variant 766":variant, "Variant 767":variant, "Variant 768":variant, "Variant 769":variant, "Variant 770":variant, "Variant 771":variant, "Variant 772":variant, "Variant 773":variant, "Variant 774":variant, "Variant 775":variant, "Variant 776":variant, "Variant 777":variant, "Variant 778":variant, "Variant 779":variant, "Variant 780":variant, "Variant 781":variant, "Variant 782":variant, "Variant 783":variant, "Variant 784":variant, "Variant 785":variant, "Variant 786":variant, "Variant 787":variant, "Variant 788":variant, "Variant 789":variant, "Variant 790":variant, "Variant 791":variant, "Variant 792":variant, "Variant 793":variant, "Variant 794":variant, "Variant 795":variant, "Variant 796":variant, "Variant 797":variant, "Variant 798":variant, "Variant 799":variant, "Variant 800":variant, "Variant 801":variant, "Variant 802":variant, "Variant 803":variant, "Variant 804":variant, "Variant 805":variant, "Variant 806":variant, "Variant 807":variant, "Variant 808":variant, "Variant 809":variant, "Variant 810":variant, "Variant 811":variant, "Variant 812":variant, "Variant 813":variant, "Variant 814":variant, "Variant 815":variant, "Variant 816":variant, "Variant 817":variant, "Variant 818":variant, "Variant 819":variant, "Variant 820":variant, "Variant 821":variant, "Variant 822":variant, "Variant 823":variant, "Variant 824":variant, "Variant 825":variant, "Variant 826":variant, "Variant 827":variant, "Variant 828":variant, "Variant 829":variant, "Variant 830":variant, "Variant 831":variant, "Variant 832":variant, "Variant 833":variant, "Variant 834":variant, "Variant 835":variant, "Variant 836":variant, "Variant 837":variant, "Variant 838":variant, "Variant 839":variant, "Variant 840":variant, "Variant 841":variant, "Variant 842":variant, "Variant 843":variant, "Variant 844":variant, "Variant 845":variant, "Variant 846":variant, "Variant 847":variant, "Variant 848":variant, "Variant 849":variant, "Variant 850":variant, "Variant 851":variant, "Variant 852":variant, "Variant 853":variant, "Variant 854":variant, "Variant 855":variant, "Variant 856":variant, "Variant 857":variant, "Variant 858":variant, "Variant 859":variant, "Variant 860":variant, "Variant 861":variant, "Variant 862":variant, "Variant 863":variant, "Variant 864":variant, "Variant 865":variant, "Variant 866":variant, "Variant 867":variant, "Variant 868":variant, "Variant 869":variant, "Variant 870":variant, "Variant 871":variant, "Variant 872":variant, "Variant 873":variant, "Variant 874":variant, "Variant 875":variant, "Variant 876":variant, "Variant 877":variant, "Variant 878":variant, "Variant 879":variant, "Variant 880":variant, "Variant 881":variant, "Variant 882":variant, "Variant 883":variant, "Variant 884":variant, "Variant 885":variant, "Variant 886":variant, "Variant 887":variant, "Variant 888":variant, "Variant 889":variant, "Variant 890":variant, "Variant 891":variant, "Variant 892":variant, "Variant 893":variant, "Variant 894":variant, "Variant 895":variant, "Variant 896":variant, "Variant 897":variant, "Variant 898":variant, "Variant 899":variant, "Variant 900":variant, "Variant 901":variant, "Variant 902":variant, "Variant 903":variant, "Variant 904":variant, "Variant 905":variant, "Variant 906":variant, "Variant 907":variant, "Variant 908":variant, "Variant 909":variant, "Variant 910":variant, "Variant 911":variant, "Variant 912":variant, "Variant 913":variant, "Variant 914":variant, "Variant 915":variant, "Variant 916":variant, "Variant 917":variant, "Variant 918":variant, "Variant 919":variant, "Variant 920":variant, "Variant 921":variant, "Variant 922":variant, "Variant 923":variant, "Variant 924":variant, "Variant 925":variant, "Variant 926":variant, "Variant 927":variant, "Variant 928":variant, "Variant 929":variant, "Variant 930":variant, "Variant 931":variant, "Variant 932":variant, "Variant 933":variant, "Variant 934":variant, "Variant 935":variant, "Variant 936":variant, "Variant 937":variant, "Variant 938":variant, "Variant 939":variant, "Variant 940":variant, "Variant 941":variant, "Variant 942":variant, "Variant 943":variant, "Variant 944":variant, "Variant 945":variant, "Variant 946":variant, "Variant 947":variant, "Variant 948":variant, "Variant 949":variant, "Variant 950":variant, "Variant 951":variant, "Variant 952":variant, "Variant 953":variant, "Variant 954":variant, "Variant 955":variant, "Variant 956":variant, "Variant 957":variant, "Variant 958":variant, "Variant 959":variant, "Variant 960":variant, "Variant 961":variant, "Variant 962":variant, "Variant 963":variant, "Variant 964":variant, "Variant 965":variant, "Variant 966":variant, "Variant 967":variant, "Variant 968":variant, "Variant 969":variant, "Variant 970":variant, "Variant 971":variant, "Variant 972":variant, "Variant 973":variant, "Variant 974":variant, "Variant 975":variant, "Variant 976":variant, "Variant 977":variant, "Variant 978":variant, "Variant 979":variant, "Variant 980":variant, "Variant 981":variant, "Variant 982":variant, "Variant 983":variant, "Variant 984":variant, "Variant 985":variant, "Variant 986":variant, "Variant 987":variant, "Variant 988":variant, "Variant 989":variant, "Variant 990":variant, "Variant 991":variant, "Variant 992":variant, "Variant 993":variant, "Variant 994":variant, "Variant 995":variant, "Variant 996":variant, "Variant 997":variant, "Variant 998":variant, "Variant 999":variant, "Variant 1000":variant}
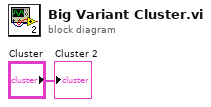
[diagram p0: block diagram]
diagram:
  "Cluster 2" <- "Cluster"
